vi "set_slider_status.vi"(8 "error in (no error)":errorcluster, 11 "DataCollectionDL090215 in":refnum<class "DataCollectionDL090215.lvclass">) -> (0 "error out":errorcluster, 3 "DataCollectionDL090215 out":refnum<class "DataCollectionDL090215.lvclass">)   [LabVIEW 2010, in "DataCollectionDL090215.lvclass"]
uses:
  DataCollectionDL090215.lvclass
  DataCollectionDL090215.lvclass/DataCollectionDL090215.ctl
  common/classes/ImageCollection/ImageCollection/ImageCollection.lvclass
  common/classes/ErrorController/ErrorController/class_data.vi
  common/classes/ErrorController/ErrorController/ErrorController.lvclass
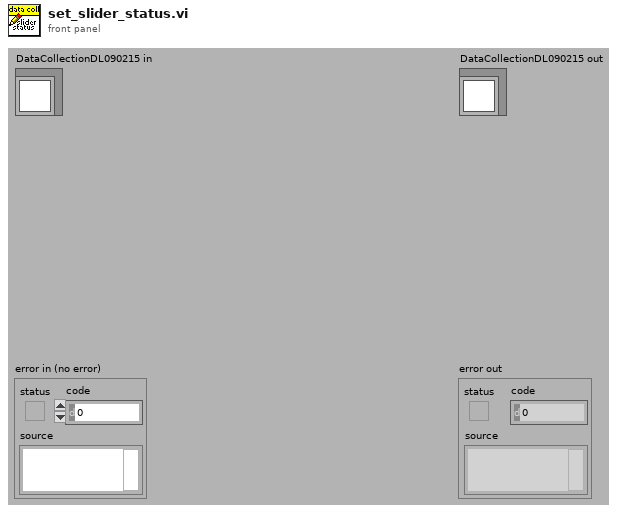
[diagram p1: front panel]
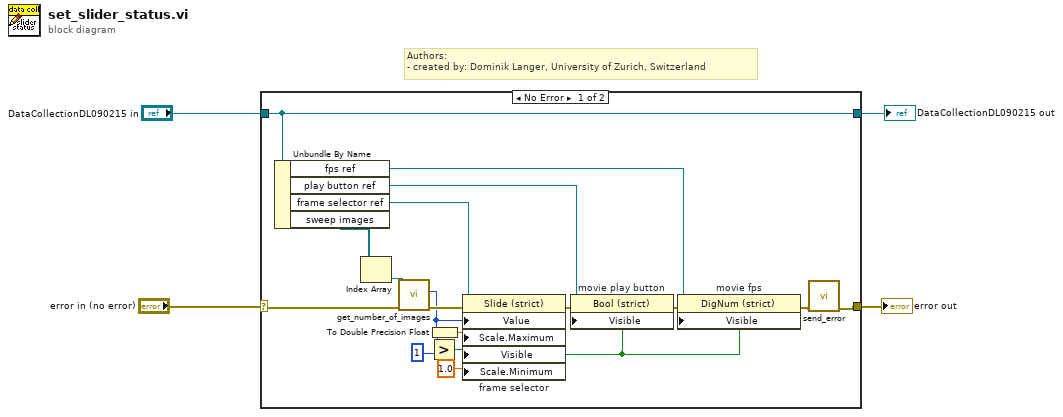
[diagram p0: block diagram]
diagram:
  # "Authors: \n- created by: Dominik Langer, University of Zurich, Switzerland"
  n1 = case shown="No Error" "error in (no error)" {
    selector: "error in (no error)" -> [w9 w23]
    tunnel: [w8 w23] -> w3
    tunnel: [w11 w22] -> w1
    tunnel: "DataCollectionDL090215 in" -> [w11 w22]
    frame No Error {
      n2 = Unbundle By Name(w11) -> ("fps ref"=w7:refnum<vi>, "play button ref"=w6:refnum<vi>, "frame selector ref"=w5:refnum<vi>, "sweep images"=w10:refnum<class "ImageCollection.lvclass">[])
      n3 = Index Array(array=w10) -> (element=w17:refnum<class "ImageCollection.lvclass">)  [unwired: 1 in]
      n4 = call-dynamic "get_number_of_images.vi"("error in (no error)"=w9, "ImageCollection in"=w17) -> ("error out"=w18:errorcluster, "size"=w16:i32)  [unwired: 8 out]
      n5 = Greater?(x=w16, y=1) -> (0:w12:bool)
      n6 = To Double Precision Float(number=w16) -> (double precision float=w19:dbl)
      n7 = property on="frame selector" class="Slide (strict)"(reference=w5, error in=w18, "Value"=w16, "Scale.Maximum"=w19, "Visible"=w12, "Scale.Minimum"=1.0) -> (error out=w15:errorcluster)  [unwired: 1 out]
      n8 = property on="movie play button" class="Bool (strict)"(reference=w6, error in=w15, "Visible"=w12) -> (error out=w14:errorcluster)  [unwired: 1 out]
      n9 = property on="movie fps" class="DigNum (strict)"(reference=w7, error in=w14, "Visible"=w12) -> (error out=w13:errorcluster)  [unwired: 1 out]
      n10 = call "send_error.vi"("error in (no error)"=w13) -> ("error out"=w8:errorcluster)  [unwired: 10 in]
    }
    frame Error {
    }
  }
  "error out" <- w3
  "DataCollectionDL090215 out" <- w1
